vi "Open DQMH Request Message Diagram QD.vi"(6 "Variant in":variant, 7 "Shift Pressed?":bool, 8 "error in (no error)":errorcluster, 10 "QD Combo Box Ref":refnum<vi>, 11 "QD Launch VI Ref":refnum<vi>) -> (0 "error out":errorcluster, 4 "Variant out":variant)   [LabVIEW 2017]
doc: "Quick Drop Ctrl-Key Shortcut (CTRL-K by default) to quickly open the Message Diagram of the Message Handling Loop within the DQMH Module Main VI.\n\nBSD 3-Clause License\n\nCopyright (c) 2022, Neosoft Technologies Inc\nAll rights reserved.\n\nRedistribution and use in source and binary forms, with or without\nmodification, are permitted provided that the following conditions are met:\n\n1. Redistributions of source code must retain the above copyright notice, this\n list of conditions and the following disclaimer.\n\n2. Redistributions in binary form must reproduce the above copyright notice,\n this list of conditions and the following disclaimer in the documentation\n and/or other materials provided with the distribution.\n\n3. Neither the name of the copyright holder nor the names of its\n contributors may be used to endorse or promote products derived from\n this software without specific prior written permission.\n\nTHIS SOFTWARE IS PROVIDED BY THE COPYRIGHT HOLDERS AND CONTRIBUTORS \"AS IS\"\nAND ANY EXPRESS OR IMPLIED WARRANTIES, INCLUDING, BUT NOT LIMITED TO, THE\nIMPLIED WARRANTIES OF MERCHANTABILITY AND FITNESS FOR A PARTICULAR PURPOSE ARE\nDISCLAIMED. IN NO EVENT SHALL THE COPYRIGHT HOLDER OR CONTRIBUTORS BE LIABLE\nFOR ANY DIRECT, INDIRECT, INCIDENTAL, SPECIAL, EXEMPLARY, OR CONSEQUENTIAL\nDAMAGES (INCLUDING, BUT NOT LIMITED TO, PROCUREMENT OF SUBSTITUTE GOODS OR\nSERVICES; LOSS OF USE, DATA, OR PROFITS; OR BUSINESS INTERRUPTION) HOWEVER\nCAUSED AND ON ANY THEORY OF LIABILITY, WHETHER IN CONTRACT, STRICT LIABILITY,\nOR TORT (INCLUDING NEGLIGENCE OR OTHERWISE) ARISING IN ANY WAY OUT OF THE USE\nOF THIS SOFTWARE, EVEN IF ADVISED OF THE POSSIBILITY OF SUCH DAMAGE.\n\nDefault Shortcut - [k]"
uses:
  vi.lib/Neosoft Technologies Inc/Open-DQMH-Request-Message-Diagram/Open DQMH Request Message Diagram.lvlib
panel:
  in  "Undo Name":string="Quick Drop Keyboard Shortcut"
  # "Do not change the connector pane of this VI.\n\nSee the block diagram for directions on how to use this template."
  # "Specify the name of the Undo transaction"
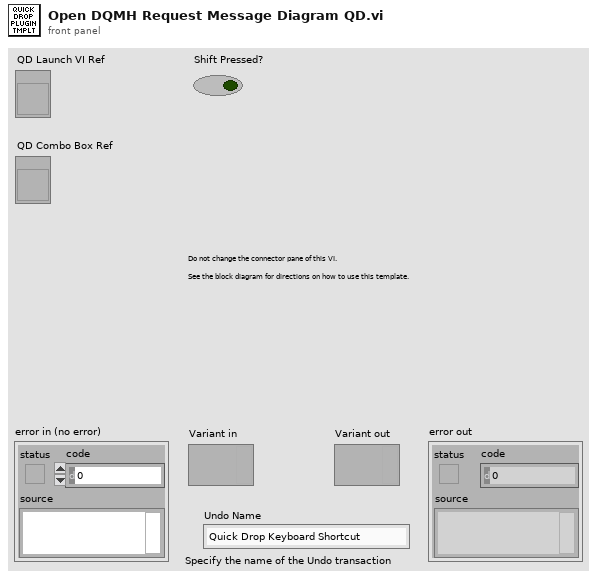
[diagram p1: front panel]
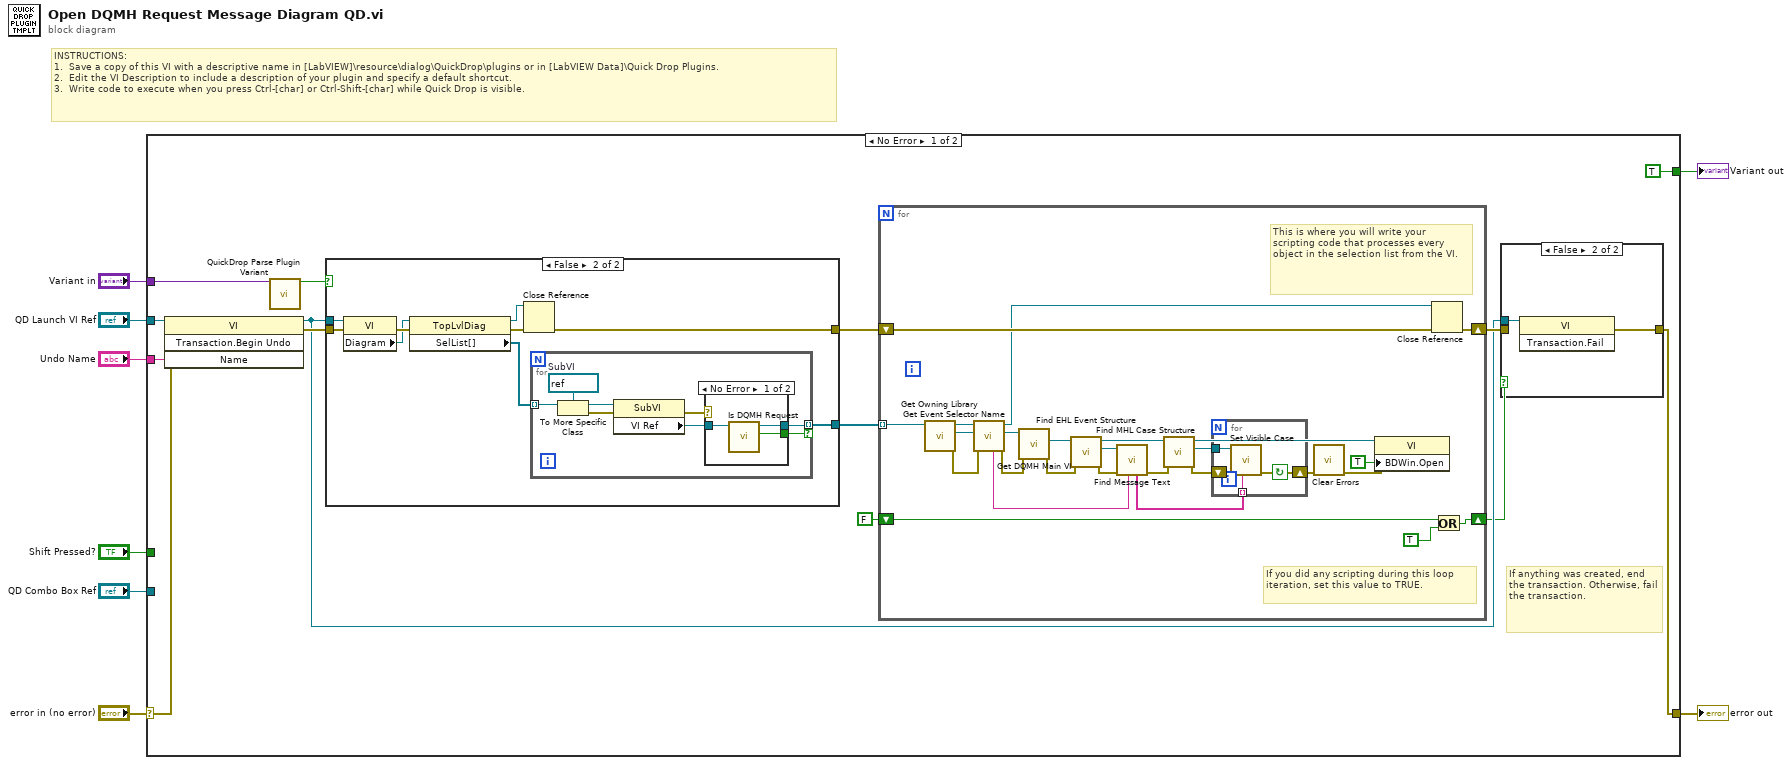
[diagram p0: block diagram]
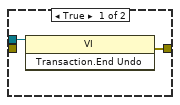
[diagram p2: hidden frame]
diagram:
  # "INSTRUCTIONS:\n1.  Save a copy of this VI with a descriptive name in [LabVIEW]\\resource\\dialog\\QuickDrop\\plugins or in [LabVIEW Data]\\Quick Drop Plugins.\n2.  Edit the VI Description to include a description of your plugin and specify a default shortcut. \n3.  Write code to execute when you press Ctrl-[char] or Ctrl-Shift-[char] while Quick Drop is visible."
  n1 = case shown="No Error" "error in (no error)" {
    selector: "error in (no error)" -> [w21 w78]
    tunnel: [w15 w78] -> w7
    tunnel: "QD Launch VI Ref" -> [w20 _]
    tunnel: "Shift Pressed?" -> [_ _]
    tunnel: "QD Combo Box Ref" -> [_ _]
    tunnel: "Variant in" -> [w22 _]
    tunnel: "Undo Name" -> [w19 _]
    tunnel: [TRUE _] -> w1
    frame No Error {
      # "If anything was created, end the transaction. Otherwise, fail the transaction."
      n2 = invoke class="VI" method="Transaction.Begin Undo"(reference=w20, error in=w21, "Name"=w19) -> (reference out=w12:refnum<vi>, error out=w16:errorcluster)  [unwired: 1 in, 2 out]
      n3 = call <vilib>:"QuickDrop Parse Plugin Variant.vi"("QDKS Variant in"=w22) -> ("QD Launch VI Panel?"=w17:bool)  [unwired: 12 in, 2 out]
      n4 = case shown="False" w17 {
        tunnel: w16 -> [w57 w66]
        tunnel: w12 -> [_ w65]
        tunnel: [w57 w60] -> w14
        tunnel: [_ w58] -> w9
        frame True {
        }
        frame False {
          n5 = property class="VI"(reference=w65, error in=w66) -> (error out=w64:errorcluster, "Diagram"=w63:refnum<vi>)  [unwired: 1 out]
          n6 = property class="TopLvlDiag"(reference=w63, error in=w64) -> (reference out=w61:refnum<vi>, error out=w62:errorcluster, "SelList[]"=w59:refnum<vi>[])
          n7 = Close Reference(reference=w61, error in (no error)=w62) -> (error out=w60:errorcluster)
          n8 = for {
            tunnel: w59 -> [w73] mode=indexing
            tunnel: [w67] -> w58 mode=indexing if=w72
            w74 = refnum<vi> refnum  # SubVI
            n9 = To More Specific Class(target class=w74, reference=w73) -> (specific class reference=w71:refnum<vi>, error out=w70:errorcluster)  [unwired: 1 in]
            n10 = property class="SubVI"(reference=w71, error in=w70) -> (error out=w69:errorcluster, "VI Ref"=w68:refnum<vi>)  [unwired: 1 out]
            n11 = case shown="No Error" w69 {
              tunnel: [w75 _] -> w72
              tunnel: w68 -> [w77 _]
              tunnel: [w76 _] -> w67
              frame No Error {
                n12 = call "Is DQMH Request.vi"("VI in"=w77) -> ("Is a DQMH Request"=w75:bool, "VI out"=w76:refnum<vi>)  [unwired: 8 in, 1 out]
              }
              frame Error {
              }
            }
          }
        }
      }
      n13 = for {
        shift-right: [w44] -> w13
        shift-left: w14 -> [w45]
        shift-right: [w47] -> w10
        shift-left: FALSE -> [w48]
        tunnel: w9 -> [w39] mode=indexing
        # "This is where you will write your scripting code that processes every object in the selection list from the VI."
        # "If you did any scripting during this loop iteration, set this value to TRUE."
        n14 = call "Get Owning Library.vi"("VI in"=w39) -> ("error out"=w41:errorcluster, "Owning Library"=w43:refnum<vi>, "VI out"=w42:refnum<vi>)  [unwired: 7 in, 1 out]
        n15 = call "Get Event Selector Name.vi"("error in (no error)"=w41, "Library Ref in"=w43, "VI Ref in"=w42) -> ("error out"=w31:errorcluster, "Library Ref out"=w40:refnum<vi>, "VI Ref out"=w25:refnum<vi>, "Event Selector Name"=w36:string)  [unwired: 5 in]
        n16 = call "Get DQMH Main VI.vi"("error in (no error)"=w31, "Library Ref in"=w40) -> ("error out"=w32:errorcluster, "Main VI Ref"=w38:refnum<vi>)  [unwired: 7 in, 1 out]
        n17 = call "Find EHL Event Structure.vi"("error in (no error)"=w32, "VI Ref in"=w38) -> ("error out"=w33:errorcluster, "EHL Event Structure"=w37:refnum<vi>, "VI Ref out"=w35:refnum<vi>)  [unwired: 6 in, 1 out]
        n18 = call "Find Message Text.vi"("Event Selector Name"=w36, "error in (no error)"=w33, "EventStructure in"=w37) -> ("error out"=w34:errorcluster, "Message Text"=w24:string[])  [unwired: 7 in]
        n19 = call "Find MHL Case Structure.vi"("error in (no error)"=w34, "VI Ref in"=w35) -> ("error out"=w28:errorcluster, "MHL Case Structure"=w30:refnum<vi>, "VI Ref out"=w29:refnum<vi>)  [unwired: 6 in, 1 out]
        n20 = for {
          tunnel: w30 -> [w52]
          tunnel: w24 -> [w50] mode=indexing
          shift-right: [w49] -> w27
          shift-left: w28 -> [w51]
          stop <- w49 continue-if-true
          n21 = call "Set Visible Case.vi"("Message Text"=w50, "error in (no error)"=w51, "CaseStructure in"=w52) -> ("error out"=w49:errorcluster)  [unwired: 8 in]
        }
        n22 = call <vilib>:"Clear Errors.vi"("error in (no error)"=w27) -> ("error out"=w23:errorcluster)  [unwired: 5 in, 1 out]
        n23 = property class="VI"(reference=w29, error in=w23, "BDWin.Open"=TRUE ("Block Diagram Window:Open")) -> ()  [unwired: 2 out]
        n24 = Close Reference(reference=w25, error in (no error)=w45) -> (error out=w44:errorcluster)
        n25 = Or(x=w48, y=TRUE ("x")) -> (x .or. y?=w47:bool)
      }
      n26 = case shown="False" w10 {
        tunnel: w12 -> [w53 w55]
        tunnel: [w54 w56] -> w15
        tunnel: w13 -> [_ _]
        frame True {
          n27 = invoke class="VI" method="Transaction.End Undo"(reference=w53) -> (error out=w54:errorcluster)  [unwired: 2 in, 2 out]
        }
        frame False {
          n28 = invoke class="VI" method="Transaction.Fail"(reference=w55) -> (error out=w56:errorcluster)  [unwired: 2 in, 2 out]
        }
      }
    }
    frame Error {
    }
  }
  "error out" <- w7
  "Variant out" <- w1
